vi "var_master.vi"(6 "generic settings":T1={"generic cmd"="", "upper_limit"=5.0, "lower limit"=0.05, "format"="%#.8g"} {"upper_limit" format="%#_13g"}, 8 "error IN":errorcluster, 10 "value IN":dbl, 11 "config":T2={"hardware"=enum."wait (s)", "options"="", "repeats"=1, "loops"=1, "VISA"="", "override_VISA"=FALSE} {"loops" min=1; "repeats" min=1}) -> (0 "error OUT":errorcluster, 1 "value OUT":dbl)   [LabVIEW 2017]
uses:
  tools/core/var_config.ctl
  var_list.ctl
  tools/core/generic_config.ctl
  tools/tools.lvlib
panel:
  # "Some -- but not all -- of \nthe hardware subVIs accept \nthe VISA resource input \nspecified in `config`.\n\nIf checked, this can be used to \noverride the subVI's default\nVISA resource."
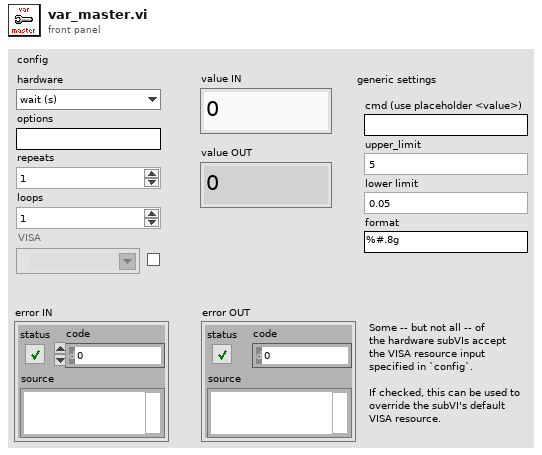
[diagram p1: front panel]
types:
  T1 = typedef "tools.lvlib/generic_config.ctl" = cluster{"generic cmd":string, "upper_limit":dbl, "lower limit":dbl, "format":string}
  T2 = typedef "tools.lvlib/var_config.ctl" = cluster{"hardware":T3, "options":string, "repeats":i32, "loops":i32, "VISA":refnum<visa-resource-name>, "override_VISA":bool}
  T3 = typedef "var_list.ctl" = enum16{"none", "AO voltage (V)", "delay (s)", "generic", "microwaves (GHz)", "radiant (nm)", "radiant thg (nm)", "sirah (nm)", "sirah_shg (nm)", "tenma voltage (V)", "wait (s)", "wf_freq (Hz)", "wf_amp (V)", "wf_amp_multi (V)", "wf_offset (V)", "wf_low_level (V)", "wf_high_level (V)", "wf_period (s)", "wf_pulse_width (s)", "wf_sample_rate (Sa/s)", "wf_multi_amp", "wf_multi_freq", "wf_arb_4chan", "WS7 setpoint (nm)"}
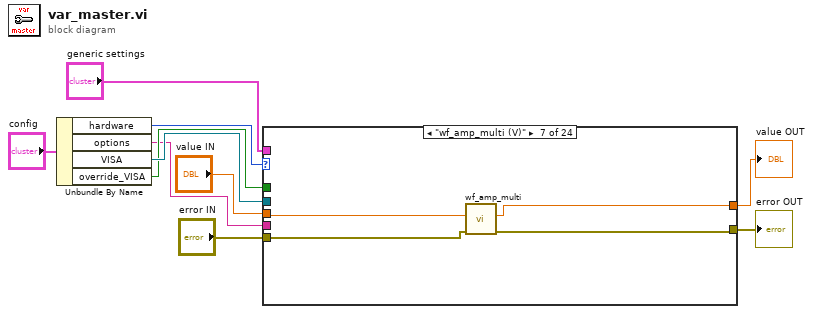
[diagram p0: block diagram]
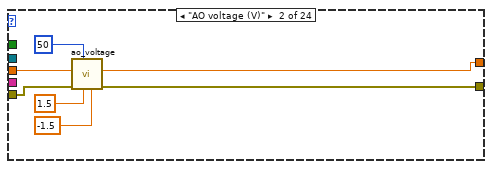
[diagram p3: hidden frame]
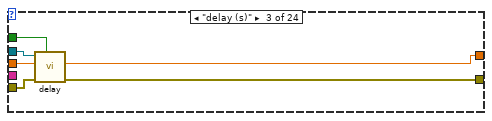
[diagram p4: hidden frame]
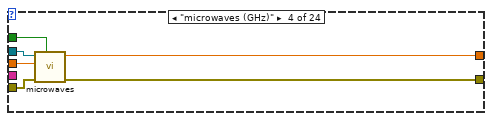
[diagram p5: hidden frame]
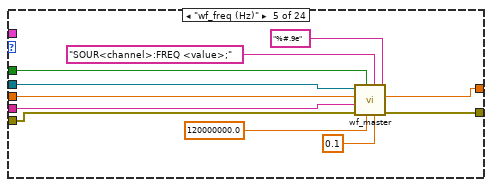
[diagram p6: hidden frame]
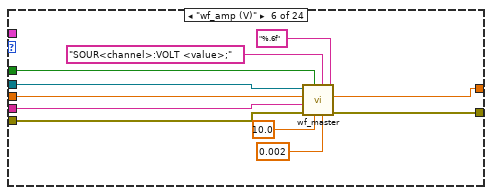
[diagram p7: hidden frame]
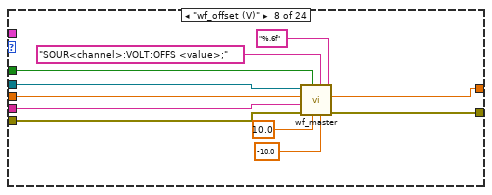
[diagram p8: hidden frame]
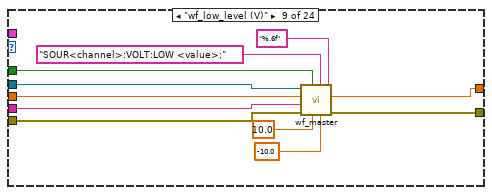
[diagram p9: hidden frame]
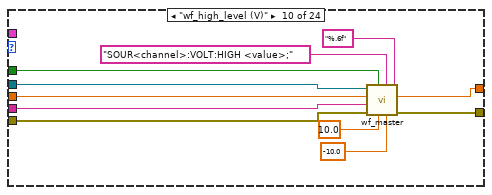
[diagram p10: hidden frame]
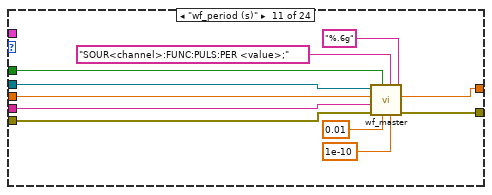
[diagram p11: hidden frame]
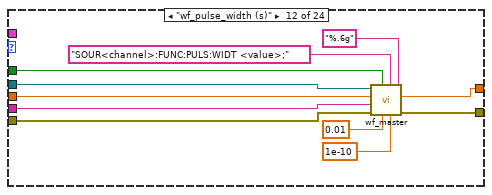
[diagram p12: hidden frame]
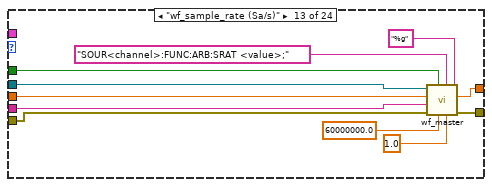
[diagram p13: hidden frame]
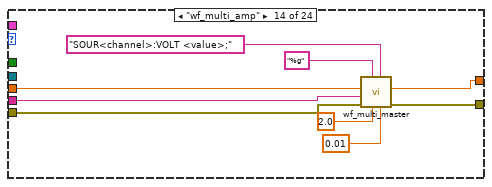
[diagram p14: hidden frame]
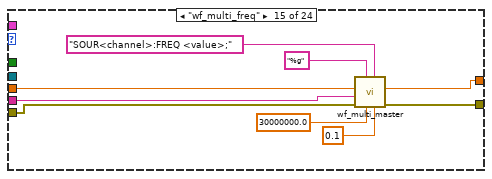
[diagram p15: hidden frame]
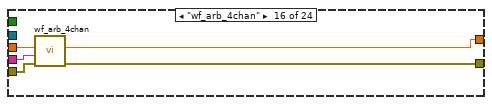
[diagram p16: hidden frame]
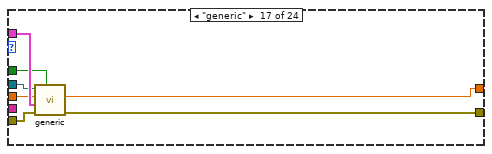
[diagram p17: hidden frame]
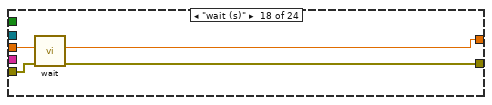
[diagram p18: hidden frame]
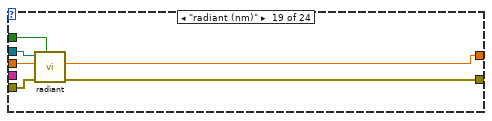
[diagram p19: hidden frame]
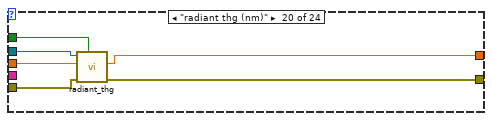
[diagram p20: hidden frame]
diagram:
  n1 = Unbundle By Name("config") -> ("hardware"=w5:T3, "options"=w2:string, "VISA"=w4:refnum<visa-resource-name>, "override_VISA"=w3:bool)
  n2 = case shown="\"wf_amp_multi (V)\"" w5 {
    tunnel: "error IN" -> [w12 w19 w25 w31 w41 w49 w57 w68 w79 w90 w97 w112 w123 w132 w141 w146 w153 w157 w162 w169 w170 w177 w181 w187]
    tunnel: [w12 w18 w24 w30 w42 w50 w56 w67 w76 w89 w100 w111 w122 w130 w139 w145 w152 w156 w161 w168 w171 w176 w180 w186] -> w9
    tunnel: [w11 w14 w23 w29 w40 w51 w55 w66 w75 w88 w99 w110 w121 w131 w140 w144 w151 w155 w160 w167 w172 w175 w178 w185] -> w8
    tunnel: "value IN" -> [w11 w13 w20 w28 w33 w45 w54 w58 w71 w80 w91 w103 w115 w124 w133 w143 w147 w154 w163 w166 w173 w174 w179 w184]
    tunnel: w4 -> [_ _ w22 w27 w34 w46 _ w60 w70 w82 w94 w104 w113 _ _ _ w149 _ w158 w165 _ _ _ w183]
    tunnel: w3 -> [_ _ w21 w26 w35 w43 _ w61 w72 w83 w95 w105 w116 _ _ _ w148 _ w159 w164 _ _ _ w182]
    tunnel: w2 -> [_ _ _ _ w32 w47 _ w59 w69 w81 w92 w102 w114 w125 w134 w142 _ _ _ _ _ _ _ _]
    tunnel: "generic settings" -> [_ _ _ _ _ _ _ _ _ _ _ _ _ _ _ _ w150 _ _ _ _ _ _ _]
    frame "none", Default {
    }
    frame "AO voltage (V)" {
      n3 = call "ao_voltage.vi"("lower limit"=-1.5, "upper limit"=1.5, "hold (ms)"=u32 50 ("delay (ms)"), "error in"=w19, "value"=w13) -> ("error out"=w18:errorcluster, "value out"=w14:dbl)  [unwired: 5 in]
    }
    frame "delay (s)" {
      n4 = call "delay.vi"("override"=w21, "error in (no error)"=w25, "delay (s)"=w20, "VISA IN"=w22) -> ("error out"=w24:errorcluster, "value out"=w23:dbl)  [unwired: 6 in]
    }
    frame "microwaves (GHz)" {
      n5 = call "microwaves.vi"("override"=w26, "error in (no error)"=w31, "frequency (GHz)"=w28, "VISA IN"=w27) -> ("error out"=w30:errorcluster, "value out"=w29:dbl)  [unwired: 6 in]
    }
    frame "wf_freq (Hz)" {
      n6 = call "wf_master.vi"("format"="%#.9e" ("value format"), "lower limit"=0.1, "template"="SOUR<channel>:FREQ <value>;", "upper limit"=120000000.0, "override"=w35, "error in (no error)"=w41, "options"=w32, "value"=w33, "VISA IN"=w34) -> ("error out"=w42:errorcluster, "value out"=w40:dbl)  [unwired: 1 in]
    }
    frame "wf_amp (V)" {
      n7 = call "wf_master.vi"("format"="%.6f" ("value format"), "lower limit"=0.002, "template"="SOUR<channel>:VOLT <value>;", "upper limit"=10.0, "override"=w43, "error in (no error)"=w49, "options"=w47, "value"=w45, "VISA IN"=w46) -> ("error out"=w50:errorcluster, "value out"=w51:dbl)  [unwired: 1 in]
    }
    frame "wf_amp_multi (V)" {
      n8 = call "wf_amp_multi.vi"("error in"=w57, "value"=w54) -> ("error out"=w56:errorcluster, "value out"=w55:dbl)  [unwired: 8 in]
    }
    frame "wf_offset (V)" {
      n9 = call "wf_master.vi"("format"="%.6f" ("value format"), "lower limit"=-10.0, "template"="SOUR<channel>:VOLT:OFFS <value>;", "upper limit"=10.0, "override"=w61, "error in (no error)"=w68, "options"=w59, "value"=w58, "VISA IN"=w60) -> ("error out"=w67:errorcluster, "value out"=w66:dbl)  [unwired: 1 in]
    }
    frame "wf_low_level (V)" {
      n10 = call "wf_master.vi"("format"="%.6f" ("value format"), "lower limit"=-10.0, "template"="SOUR<channel>:VOLT:LOW <value>;", "upper limit"=10.0, "override"=w72, "error in (no error)"=w79, "options"=w69, "value"=w71, "VISA IN"=w70) -> ("error out"=w76:errorcluster, "value out"=w75:dbl)  [unwired: 1 in]
    }
    frame "wf_high_level (V)" {
      n11 = call "wf_master.vi"("format"="%.6f" ("value format"), "lower limit"=-10.0, "template"="SOUR<channel>:VOLT:HIGH <value>;", "upper limit"=10.0, "override"=w83, "error in (no error)"=w90, "options"=w81, "value"=w80, "VISA IN"=w82) -> ("error out"=w89:errorcluster, "value out"=w88:dbl)  [unwired: 1 in]
    }
    frame "wf_period (s)" {
      n12 = call "wf_master.vi"("format"="%.6g" ("value format"), "lower limit"=1e-10, "template"="SOUR<channel>:FUNC:PULS:PER <value>;", "upper limit"=0.01, "override"=w95, "error in (no error)"=w97, "options"=w92, "value"=w91, "VISA IN"=w94) -> ("error out"=w100:errorcluster, "value out"=w99:dbl)  [unwired: 1 in]
    }
    frame "wf_pulse_width (s)" {
      n13 = call "wf_master.vi"("format"="%.6g" ("value format"), "lower limit"=1e-10, "template"="SOUR<channel>:FUNC:PULS:WIDT <value>;", "upper limit"=0.01, "override"=w105, "error in (no error)"=w112, "options"=w102, "value"=w103, "VISA IN"=w104) -> ("error out"=w111:errorcluster, "value out"=w110:dbl)  [unwired: 1 in]
    }
    frame "wf_sample_rate (Sa/s)" {
      n14 = call "wf_master.vi"("format"="%g" ("value format"), "lower limit"=1.0, "template"="SOUR<channel>:FUNC:ARB:SRAT <value>;", "upper limit"=60000000.0, "override"=w116, "error in (no error)"=w123, "options"=w114, "value"=w115, "VISA IN"=w113) -> ("error out"=w122:errorcluster, "value out"=w121:dbl)  [unwired: 1 in]
    }
    frame "wf_multi_amp" {
      n15 = call "wf_multi_master.vi"("lower limit"=0.01, "template"="SOUR<channel>:VOLT <value>;", "upper limit"=2.0, "format"="%g", "error in (no error)"=w132, "options (rescale)"=w125, "value"=w124) -> ("error out"=w130:errorcluster, "value out"=w131:dbl)  [unwired: 3 in]
    }
    frame "wf_multi_freq" {
      n16 = call "wf_multi_master.vi"("lower limit"=0.1, "template"="SOUR<channel>:FREQ <value>;", "upper limit"=30000000.0, "format"="%g", "error in (no error)"=w141, "options (rescale)"=w134, "value"=w133) -> ("error out"=w139:errorcluster, "value out"=w140:dbl)  [unwired: 3 in]
    }
    frame "wf_arb_4chan" {
      n17 = call "wf_arb_4chan.vi"("error in (no error)"=w146, "options (amp)"=w142, "w"=w143) -> ("error out"=w145:errorcluster, "value OUT"=w144:dbl)  [unwired: 7 in]
    }
    frame "generic" {
      n18 = call "generic.vi"("override"=w148, "error in (no error)"=w153, "generic settings"=w150, "Value"=w147, "VISA IN"=w149) -> ("error out"=w152:errorcluster, "value out"=w151:dbl)  [unwired: 4 in, 1 out]
    }
    frame "wait (s)" {
      n19 = call "wait.vi"("error in (no error)"=w157, "wait (s)"=w154) -> ("error out"=w156:errorcluster, "value out"=w155:dbl)  [unwired: 8 in]
    }
    frame "radiant (nm)" {
      n20 = call "radiant.vi"("override"=w159, "error in (no error)"=w162, "WL (nm)"=w163, "VISA IN"=w158) -> ("error out"=w161:errorcluster, "value out"=w160:dbl)  [unwired: 5 in, 1 out]
    }
    frame "radiant thg (nm)" {
      n21 = call "radiant_thg.vi"("override"=w164, "error in (no error)"=w169, "WL (nm)"=w166, "VISA IN"=w165) -> ("error out"=w168:errorcluster, "value out"=w167:dbl)  [unwired: 5 in, 1 out]
    }
    frame "WS7 setpoint (nm)" {
      n22 = call "WS7_setpoint.vi"("error in (no error)"=w170, "set point"=w173) -> ("error out"=w171:errorcluster, "set point (out)"=w172:dbl)  [unwired: 7 in, 1 out]
    }
    frame "sirah (nm)" {
      n23 = call "sirah.vi"("error in (no error)"=w177, "wavelength (nm)"=w174) -> ("error out"=w176:errorcluster, "value out"=w175:dbl)  [unwired: 7 in, 1 out]
    }
    frame "sirah_shg (nm)" {
      n24 = call "sirah_shg.vi"("error in (no error)"=w181, "wavelength (nm)"=w179) -> ("error out"=w180:errorcluster, "value out"=w178:dbl)  [unwired: 7 in, 1 out]
    }
    frame "tenma voltage (V)" {
      n25 = call "tenma_voltage.vi"("override"=w182, "error in (no error)"=w187, "voltage (V)"=w184, "VISA IN"=w183) -> ("error out"=w186:errorcluster, "value out"=w185:dbl)  [unwired: 6 in]
    }
  }
  "error OUT" <- w9
  "value OUT" <- w8
